vi "run_python.vi"() -> ()   [LabVIEW 2025]
uses:
  global_receive.vi
  <vilib>/Instr/_visa.llb/VISA Configure Serial Port (Instr).vi
panel:
  out "OK":bool
  in  "Home Button":bool
  out "error?":bool
  in  "Directive":string
  out "Terminal":string
  in  "Send":bool
  out "Baud Rate":u32=115200
  in  "stop":bool
  in  "COM Port":refnum<visa-resource-name>
  in  "Set Position (mm)":dbl[](array[numeric])
  out "Current Position":dbl[](array[numeric])
  in  "Send Position":bool
  # "Position Control - Absolute"
  # "Communication Breakdown"
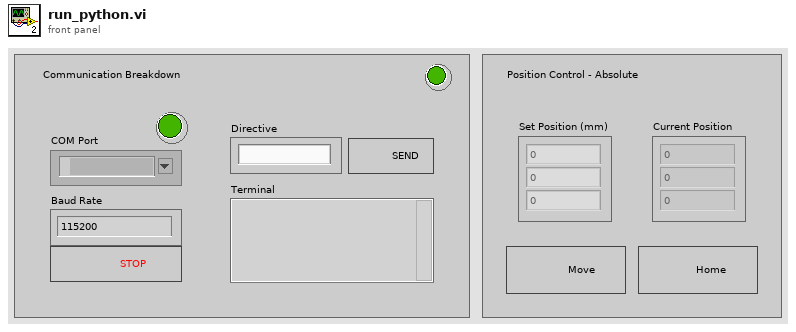
[diagram p1: front panel]
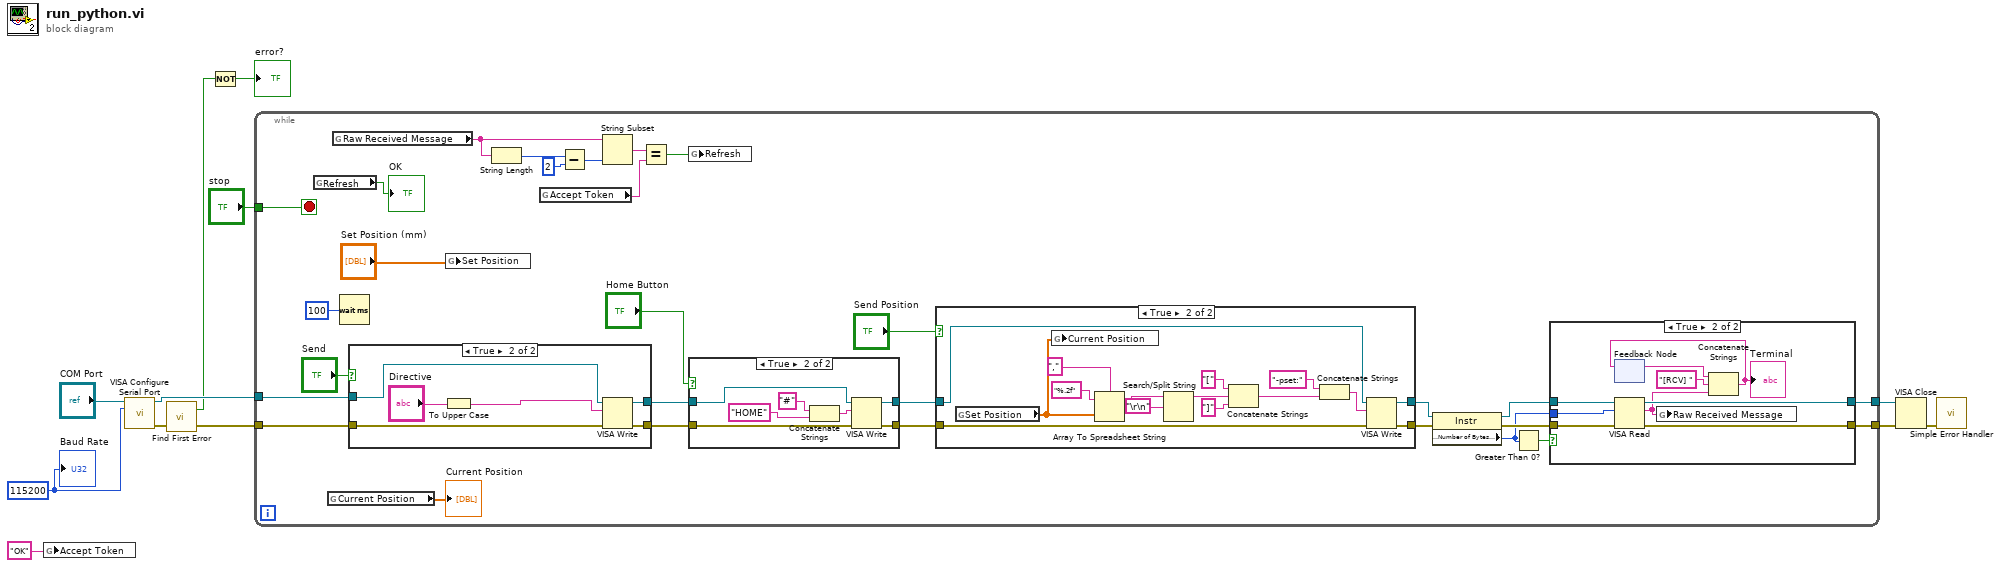
[diagram p0: block diagram]
diagram:
  w6 = u32 115200 ("Baud Rate")
  n1 = global write "global_receive.vi" "Accept Token"("OK") -> ()
  n2 = call-poly "VISA Configure Serial Port"("VISA resource name"="COM Port", "baud rate (9600)"=w6) -> ("VISA resource name out"=w12:refnum<visa-resource-name>, "error out"=w5:errorcluster)  [unwired: 12 in]
  n3 = call <vilib>:"Find First Error.vi"("error in (no error)"=w5) -> ("error out"=w4:errorcluster, "error?"=w3:bool)  [unwired: 3 in]
  n4 = Not(x=w3) -> (.not. x?=→"error?":bool)
  n5 = while {
    tunnel: w12 -> [w36]
    tunnel: w4 -> [w35]
    tunnel: [w41] -> w11
    tunnel: [w40] -> w10
    tunnel: "stop" -> [w22]
    stop <- w22 stop-if-true
    n6 = global read "global_receive.vi" "Refresh"() -> (→"OK":bool)
    n7 = global read "global_receive.vi" "Current Position"() -> (→"Current Position":dbl[])
    n8 = global read "global_receive.vi" "Raw Received Message"() -> (w17:string)
    n9 = Wait (ms)(milliseconds to wait=u32 100) -> ()  [unwired: 1 out]
    n10 = case shown="True" "Send" {
      tunnel: w36 -> [w80 w86]
      tunnel: w35 -> [w79 w85]
      tunnel: [w79 w84] -> w25
      tunnel: [w80 w83] -> w28
      frame False {
      }
      frame True {
        n11 = To Upper Case(1:"Directive") -> (0:w81:string)
        n12 = VISA Write(VISA resource name=w86, write buffer=w81, error in (no error)=w85) -> (VISA resource name out=w83:refnum<visa-resource-name>, error out=w84:errorcluster)  [unwired: 1 out]
      }
    }
    n13 = global write "global_receive.vi" "Set Position"("Set Position (mm)") -> ()
    n14 = String Length(string=w17) -> (length=w19:i32)
    n15 = global read "global_receive.vi" "Accept Token"() -> (w20:string)
    n16 = Subtract(x=w19, y=2) -> (x-y=w15:i32)
    n17 = String Subset(string=w17, length (rest)=w15) -> (substring=w16:string)  [unwired: 1 in]
    n18 = Equal?(x=w16, y=w20) -> (x = y?=w14:bool)
    n19 = global write "global_receive.vi" "Refresh"(w14) -> ()
    n20 = case shown="True" "Home Button" {
      tunnel: w28 -> [w43 w48]
      tunnel: [w43 w46] -> w27
      tunnel: [w42 w45] -> w26
      tunnel: w25 -> [w42 w47]
      frame False {
      }
      frame True {
        n21 = Concatenate Strings("#", "HOME" ("string")) -> (w50:string)
        n22 = VISA Write(VISA resource name=w48, write buffer=w50, error in (no error)=w47) -> (VISA resource name out=w46:refnum<visa-resource-name>, error out=w45:errorcluster)  [unwired: 1 out]
      }
    }
    n23 = case shown="True" "Send Position" {
      tunnel: w26 -> [w51 w67]
      tunnel: w27 -> [w52 w66]
      tunnel: [w51 w65] -> w31
      tunnel: [w52 w64] -> w30
      frame False {
      }
      frame True {
        n24 = global read "global_receive.vi" "Set Position"() -> (w53:dbl[])
        n25 = global write "global_receive.vi" "Current Position"(w53) -> ()
        n26 = Array To Spreadsheet String(delimiter (Tab)=",", array=w53, 3:"%.2f") -> (spreadsheet string=w56:string)
        n27 = Search/Split String(string=w56, search string/char (-)="\r\n") -> (substring before match=w55:string)  [unwired: 1 in, 2 out]
        n28 = Concatenate Strings("[", w55, "]") -> (w54:string)
        n29 = Concatenate Strings("-pset:", w54) -> (w62:string)
        n30 = VISA Write(VISA resource name=w66, write buffer=w62, error in (no error)=w67) -> (VISA resource name out=w64:refnum<visa-resource-name>, error out=w65:errorcluster)  [unwired: 1 out]
      }
    }
    n31 = property class="Instr"(reference=w30, error in=w31) -> (reference out=w39:refnum<visa-resource-name>, error out=w38:errorcluster, "Serial Settings:Number of Bytes at Serial Port"=w37:u32)
    n32 = Greater Than 0?(x=w37) -> (x > 0?=w34:bool)
    n33 = case shown="True" w34 {
      tunnel: w38 -> [w68 w78]
      tunnel: [w68 w77] -> w41
      tunnel: [w69 w76] -> w40
      tunnel: w39 -> [w69 w75]
      tunnel: w37 -> [_ w74]
      frame False {
      }
      frame True {
        n34 = feedback #1() -> (w71:string)  [unwired: 1 in]
        n35 = VISA Read(VISA resource name=w75, byte count=w74, error in (no error)=w78) -> (VISA resource name out=w76:refnum<visa-resource-name>, read buffer=w72:string, error out=w77:errorcluster)  [unwired: 1 out]
        n36 = global write "global_receive.vi" "Raw Received Message"(w72) -> ()
        n37 = Concatenate Strings(w71, "[RCV] ", w72) -> (w70:string)
        "Terminal" <- w70
        n38 = feedback-in #1(w70) -> ()
      }
    }
  }
  n39 = VISA Close(VISA resource name=w10, error in (no error)=w11) -> (error out=w8:errorcluster)
  n40 = call <vilib>:"Simple Error Handler.vi"("error in (no error)"=w8) -> ()  [unwired: 4 in, 5 out]
  "Baud Rate" <- w6
